vi "CreateOld SerializableDataTypedef.vi"(4 "SerializableData_v2.ctl":path, 6 "SerializableData.ctl path":path, 7 "New BlueSerializableVersion":u16, 8 "error in (no error)":errorcluster, 10 "Application":refnum<vi>, 11 "LVClassLibrary Ref":refnum<vi>) -> (0 "error out":errorcluster, 2 "Application":refnum<vi>, 3 "LVClassLibrary Ref":refnum<vi>)   [LabVIEW 2019, in "BlueSerializationScripts.lvlib"]
uses:
  BlueSerializationScripts.lvlib
  BlueSerialVirtualFolders.ctl
  <vilib>/LabVIEW Icon API/LabVIEW Icon API.lvlib
  BlueUtilityScripts/BlueUtilityScripts.lvlib
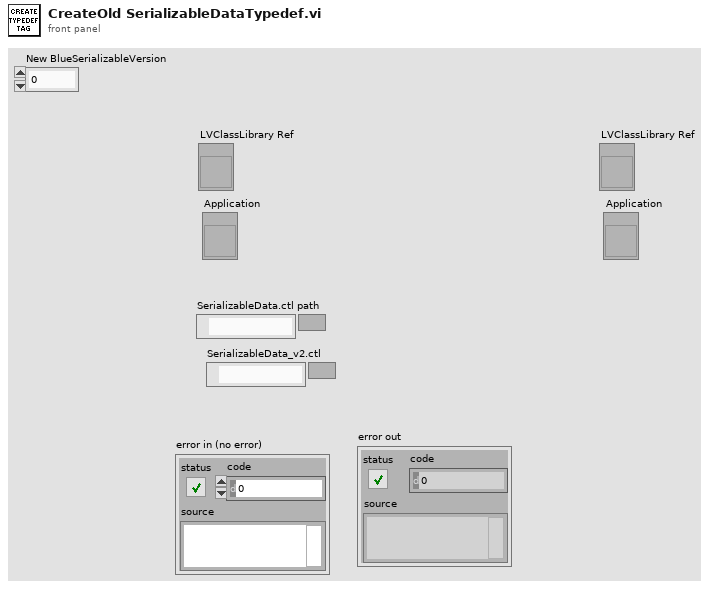
[diagram p1: front panel]
types:
  T1 = enum32{"invalid VI type", "Standard VI", "Control VI", "Global VI", "Polymorphic VI", "Configuration VI", "SubSystem", "Facade VI", "Method VI"}
  T2 = typedef "BlueSerializationScripts.lvlib/BlueSerialVirtualFolders.ctl" = enum16{"BlueSerialization", "Mutations"}
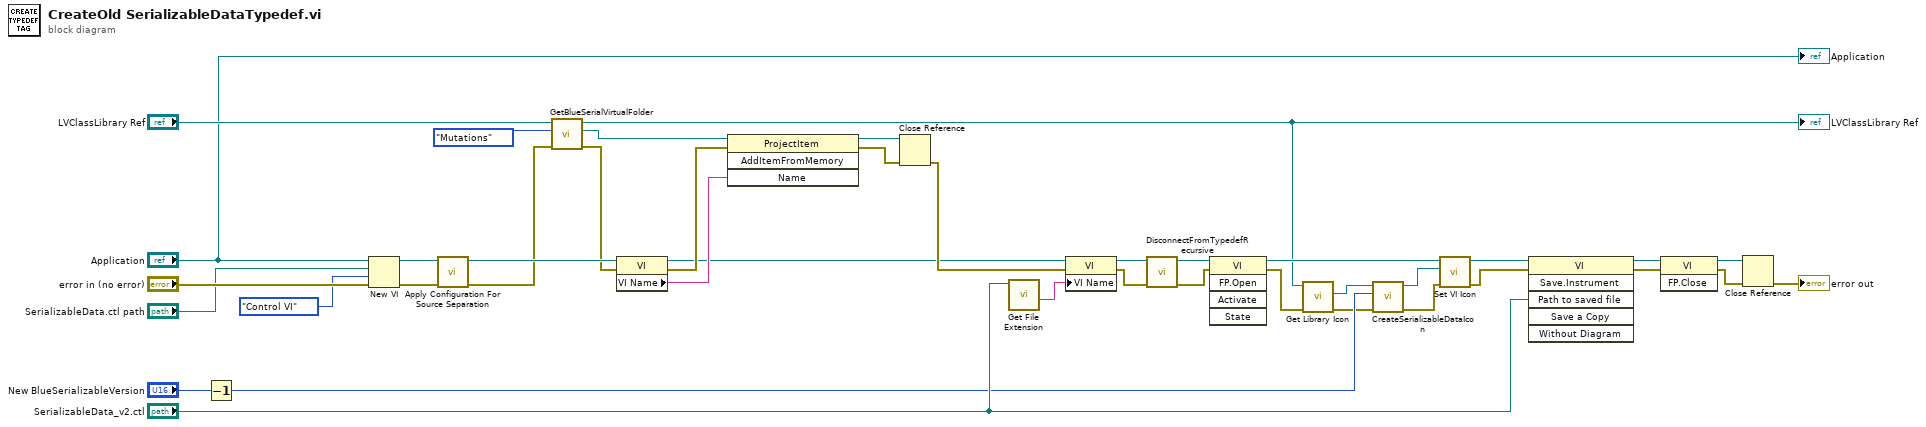
[diagram p0: block diagram]
diagram:
  n1 = Decrement(x="New BlueSerializableVersion") -> (x-1=w9:u16)
  n2 = New VI(8:"error in (no error)", 9:T1."Control VI" ("vi type (standard vi)"), 10:"SerializableData.ctl path", 11:"Application") -> (0:w19:errorcluster, 3:w18:refnum<vi>)  [unwired: 3 out]
  n3 = call <vilib>:"Apply Configuration For Source Separation.vi"("error in (no error)"=w19, "VI in"=w18) -> ("error out"=w22:errorcluster, "VI out"=w40:refnum<vi>)  [unwired: 8 in]
  n4 = call "GetBlueSerialVirtualFolder.vi"("error in (no error)"=w22, "Virtual Folder"=BlueSerialVirtualFolders."Mutations", "LVClassLibrary Ref"="LVClassLibrary Ref") -> ("error out"=w23:errorcluster, "Folder Refnum out"=w24:refnum<vi>, "LVClassLibrary Ref"=w5:refnum<vi>)  [unwired: 6 in]
  "LVClassLibrary Ref" <- w5
  n5 = property class="VI"(reference=w40, error in=w23) -> (reference out=w28:refnum<vi>, error out=w31:errorcluster, "VI Name"=w30:string)
  n6 = invoke class="ProjectItem" method="AddItemFromMemory"(reference=w24, error in=w31, "Name"=w30) -> (reference out=w32:refnum<vi>, error out=w33:errorcluster)  [unwired: 1 in, 2 out]
  n7 = Close Reference(reference=w32, error in (no error)=w33) -> (error out=w29:errorcluster)
  n8 = call <vilib>:"Get File Extension.vi"("file"="SerializableData_v2.ctl") -> ("filename without extension"=w27:string)  [unwired: 6 in, 4 out]
  n9 = property class="VI"(reference=w28, error in=w29, "VI Name"=w27) -> (reference out=w4:refnum<vi>, error out=w3:errorcluster)
  n10 = call "DisconnectFromTypedefRecursive.vi"("error in (no error)"=w3, "VI ref (typedef)"=w4) -> ("error out"=w1:errorcluster, "VI ref (typedef)"=w2:refnum<vi>)  [unwired: 8 in]
  n11 = invoke class="VI" method="FP.Open"(reference=w2, error in=w1) -> (reference out=w15:refnum<vi>, error out=w6:errorcluster)  [unwired: 3 in, 3 out]
  n12 = call <vilib>:"Get Library Icon.vi"("error in (no error)"=w6, "Library Refnum in"=w5) -> ("error out"=w7:errorcluster, "Icon"=w8:refnum<class "Icon.lvclass">)  [unwired: 7 in, 1 out]
  n13 = call "CreateSerializableDataIcon.vi"("error in (no error)"=w7, "BlueSerializableVersion"=w9, "Icon.lvclass in"=w8) -> ("error out"=w13:errorcluster, "Icon.lvlclass out"=w14:refnum<class "Icon.lvclass">)  [unwired: 6 in, 1 out]
  n14 = call <vilib>:"Set VI Icon.vi"("error in (no error)"=w13, "Icon"=w14, "VI Refnum in"=w15) -> ("error out"=w11:errorcluster, "VI Refnum out"=w12:refnum<vi>)  [unwired: 7 in]
  n15 = invoke class="VI" method="Save.Instrument"(reference=w12, error in=w11, "Path to saved file"="SerializableData_v2.ctl") -> (reference out=w39:refnum<vi>, error out=w38:errorcluster)  [unwired: 3 in, 4 out]
  n16 = invoke class="VI" method="FP.Close"(reference=w39, error in=w38) -> (reference out=w37:refnum<vi>, error out=w36:errorcluster)  [unwired: 1 in, 1 out]
  n17 = Close Reference(reference=w37, error in (no error)=w36) -> (error out=→"error out":errorcluster)
  "Application" <- "Application"
